vi "test ReadFieldWidthY.vi"(8 "error in (no error)":errorcluster, 11 "TestCase in":refnum<class "FieldTests.lvclass">) -> (0 "error out":errorcluster, 3 "TestCase out":refnum<class "FieldTests.lvclass">)   [LabVIEW 2014, in "FieldTests.lvclass"]
uses:
  FieldTests.lvclass
  SPLAT/Field Class/Field.lvclass
  <vilib>/addons/_JKI Toolkits/VI Tester/TestCase.llb/TestCase.lvclass
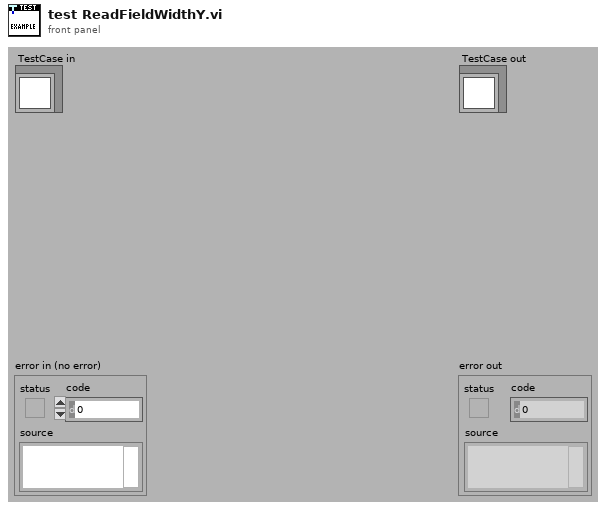
[diagram p1: front panel]
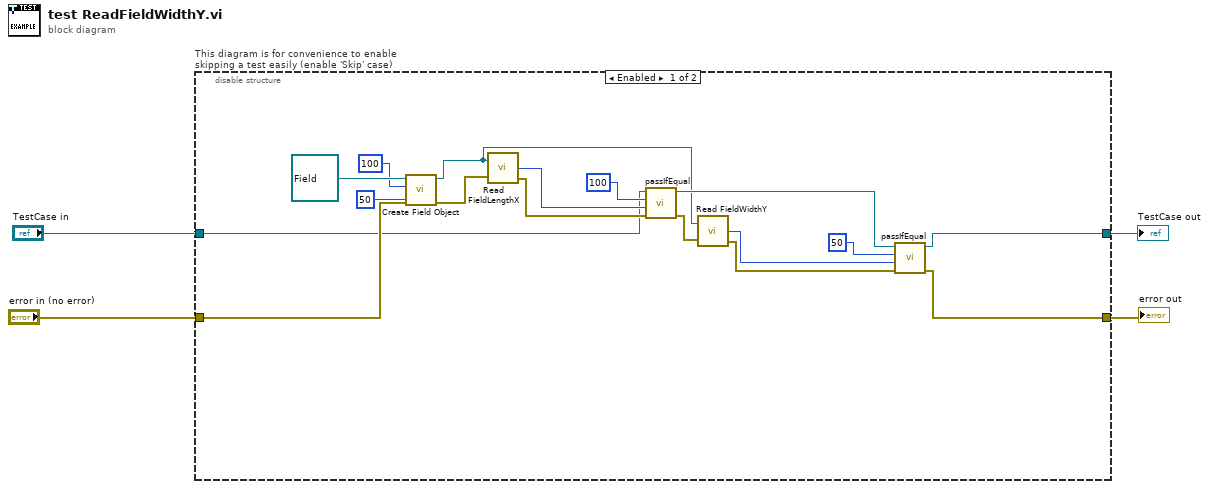
[diagram p0: block diagram]
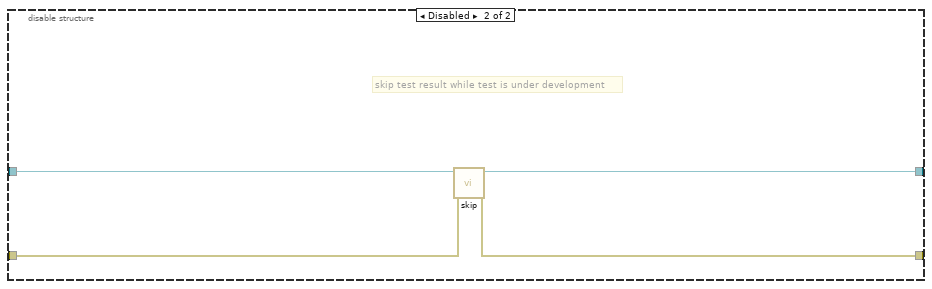
[diagram p2: hidden frame]
diagram:
  n1 = disable-structure "This diagram is for convenience to enable skipping a test easily (enable 'Skip' case)" shown="Enabled" {
    disable-tunnel: "TestCase in" -> [w7 w25]
    disable-tunnel: [w6 w23] -> w1
    disable-tunnel: [w5 w24] -> w3
    disable-tunnel: "error in (no error)" -> [w8 w22]
    frame Enabled {
      n2 = call "Create Field Object.vi"("error in (no error)"=w8, "FieldWidthY"=50, "FieldLengthX"=100, "Field in"=refnum<class "Field.lvclass"> refnum) -> ("error out"=w17:errorcluster, "Field out"=w13:refnum<class "Field.lvclass">)  [unwired: 6 in]
      n3 = call-dynamic "Read FieldLengthX.vi"("Field in"=w13, "error in (no error)"=w17) -> ("FieldLengthX"=w15:i32, "error out"=w16:errorcluster)  [unwired: 1 out]
      n4 = call-dynamic "passIfEqual.vi"("error in (no error)"=w16, "y"=w15, "x"=100 ("FieldLengthX"), "TestCase in"=w7) -> ("error out"=w12:errorcluster, "TestCase out"=w21:refnum<class "FieldTests.lvclass">)  [unwired: 6 in]
      n5 = call-dynamic "Read FieldWidthY.vi"("Field in"=w13, "error in (no error)"=w12) -> ("FieldWidthY"=w10:i32, "error out"=w11:errorcluster)  [unwired: 1 out]
      n6 = call-dynamic "passIfEqual.vi"("error in (no error)"=w11, "y"=w10, "x"=50 ("FieldWidthY"), "TestCase in"=w21) -> ("error out"=w5:errorcluster, "TestCase out"=w6:refnum<class "FieldTests.lvclass">)  [unwired: 6 in]
    }
    frame Disabled {
      # "skip test result while test is under development"
      n7 = call <vilib>:"skip.vi"("error in (no error)"=w22, "TestCase in"=w25) -> ("error out"=w24:errorcluster, "TestCase out"=w23:refnum<class "FieldTests.lvclass">)  [unwired: 8 in]
    }
  }
  "error out" <- w3
  "TestCase out" <- w1
